vi "Database Process Block Commands.vi"(8 "error in (no error)":errorcluster, 10 "Database Commands (\"\")":string, 11 "Connection Refnum":T1) -> (0 "error out":errorcluster, 3 "Connection Refnum":T1)   [LabVIEW 2011]
uses:
  Summitek EXT/ODBC/SQL Controls/Connection Refnum.ctl
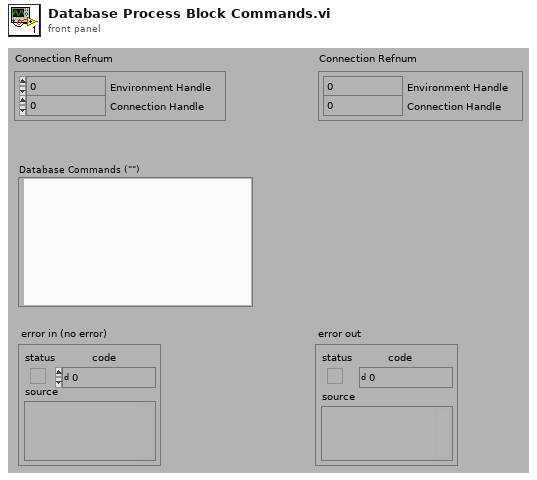
[diagram p1: front panel]
types:
  T1 = typedef "Connection Refnum.ctl" = cluster{"Environment Handle":i32, "Connection Handle":i32}
  T2 = typedef "Statement Refnum.ctl" = cluster{"Statement Handle":i32, "Parameter Number":u16}
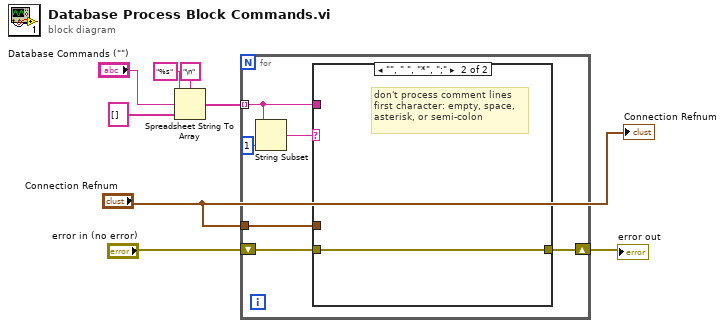
[diagram p0: block diagram]
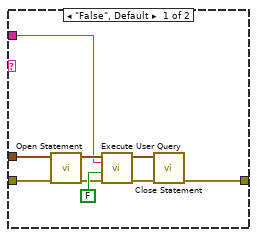
[diagram p2: hidden frame]
diagram:
  n1 = Spreadsheet String To Array(delimiter (Tab)="\n", format string="%s", spreadsheet string="Database Commands (\"\")", array type (2D Dbl)=string[] []) -> (array=w8:string[])
  n2 = for {
    tunnel: "Connection Refnum" -> [w14]
    shift-right: [w12] -> w4
    shift-left: "error in (no error)" -> [w13]
    tunnel: w8 -> [w11] mode=indexing
    n3 = String Subset(string=w11, length (rest)=1 ("length (rest)")) -> (substring=w9:string)  [unwired: 1 out]
    n4 = case shown="\"\", \" \", \"*\", \";\"" w9 {
      tunnel: w14 -> [w20 _]
      tunnel: w13 -> [w17 w24]
      tunnel: [w16 w24] -> w12
      tunnel: w11 -> [w15 _]
      frame "False", Default {
        n5 = call "Open Statement.vi"("error in (no error)"=w17, "Connection Refnum"=w20) -> ("error out"=w22:errorcluster, "Statement Refnum"=w21:T2)  [unwired: 4 out]
        n6 = call "Execute User Query.vi"("error in (no error)"=w22, "Return Data? (f)"=FALSE, "User Query"=w15, "Statement Refnum"=w21) -> ("error out"=w18:errorcluster, "Statement Refnum"=w19:T2)  [unwired: 2 out]
        n7 = call "Close Statement.vi"("error in (no error)"=w18, "Statement Refnum"=w19) -> ("error out"=w16:errorcluster)  [unwired: 5 out]
      }
      frame "", " ", "*", ";" {
        # "don't process comment lines\nfirst character: empty, space,\nasterisk, or semi-colon"
      }
    }
  }
  "error out" <- w4
  "Connection Refnum" <- "Connection Refnum"
